vi "Update from Shared Variable.vi"(7 "Force Write (F)":bool, 8 "error in (no error)":errorcluster, 10 "OPC UA server refnum in":refnum<k21>, 11 "SV Sync Tag":refnum<class "Synchronised Tag.lvclass">) -> (0 "error out":errorcluster, 2 "OPC UA server refnum out":refnum<k21>, 3 "SV Sync Tag Out":refnum<class "Synchronised Tag.lvclass">)   [LabVIEW 2016, in "Synchronised Tag.lvclass"]
doc: "Reads the latest value from the shared variable engine and updates the OPC UA server if the value has changed. Use <b>Force Write</b> to write the value whether it has changed or not."
uses:
  Synchronised Tag.lvclass
  Synchronised Tag.lvclass/Synchronised Tag.ctl
  <vilib>/OPCUA/server/Write Double.vi
  <vilib>/OPCUA/server/Write Double Array.vi
  <vilib>/OPCUA/server/Write String.vi
  <vilib>/OPCUA/server/Write String Array.vi
  <vilib>/OPCUA/server/Write Bool.vi
  <vilib>/OPCUA/server/Write Bool Array.vi
  <vilib>/OPCUA/server/Write SByte.vi
  <vilib>/OPCUA/server/Write SByte Array.vi
  <vilib>/OPCUA/server/Write Byte.vi
  <vilib>/OPCUA/server/Write Byte Array.vi
  <vilib>/OPCUA/server/Write Int16.vi
  <vilib>/OPCUA/server/Write Int16 Array.vi
  <vilib>/OPCUA/server/Write UInt16.vi
  <vilib>/OPCUA/server/Write UInt16 Array.vi
  <vilib>/OPCUA/server/Write Int32.vi
  <vilib>/OPCUA/server/Write Int32 Array.vi
  <vilib>/OPCUA/server/Write UInt32.vi
  <vilib>/OPCUA/server/Write UInt32 Array.vi
  <vilib>/OPCUA/server/Write Int64.vi
  <vilib>/OPCUA/server/Write Int64 Array.vi
  <vilib>/OPCUA/server/Write UInt64.vi
  <vilib>/OPCUA/server/Write UInt64 Array.vi
  <vilib>/OPCUA/server/Write Float.vi
  <vilib>/OPCUA/server/Write Float Array.vi
  <vilib>/OPCUA/NI OPC UA Server.lvlib
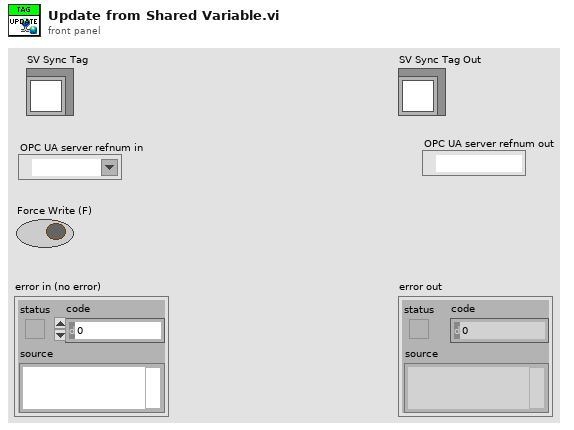
[diagram p1: front panel]
types:
  T1 = typedef "SV type.ctl" = enum16{"Boolean", "SByte", "Byte", "Int16", "UInt16", "Int32", "UInt32", "Int64", "UInt64", "Float", "Double", "String", "DateTime", "ByteString", "Array of Boolean", "Array of SByte", "Array of Byte", "Array of Int16", "Array of UInt16", "Array of Int32", "Array of UInt32", "Array of Int64", "Array of UInt64", "Array of Float", "Array of Double", "Array of String", "Array of DateTime", "Array of ByteString", "Unsupported"}
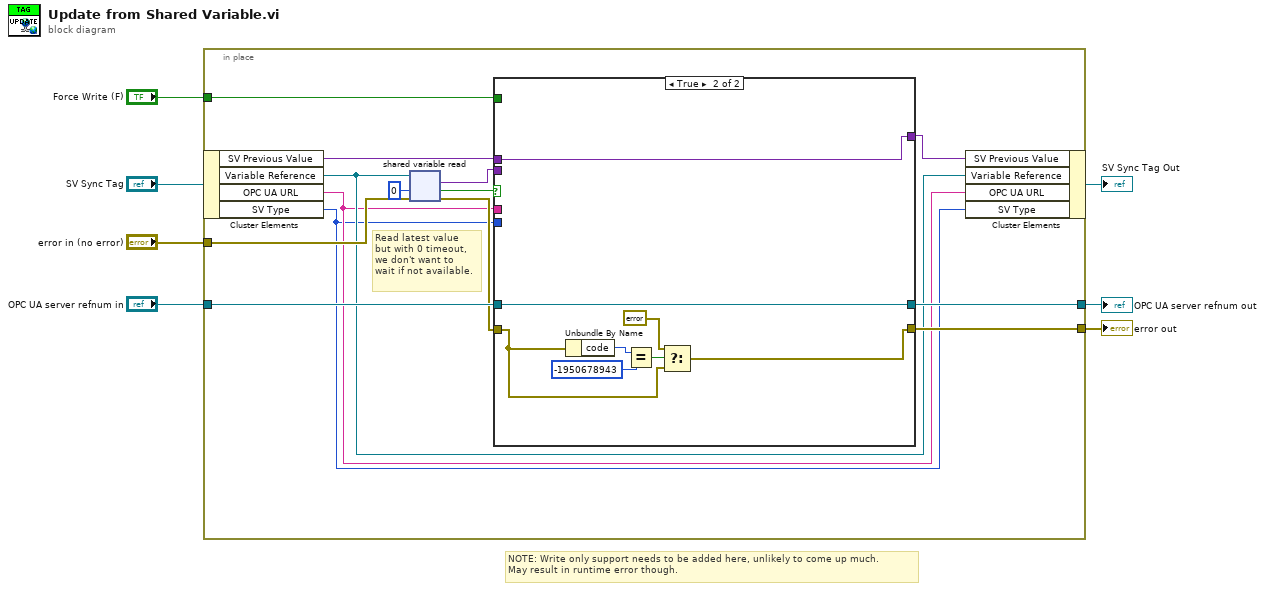
[diagram p0: block diagram]
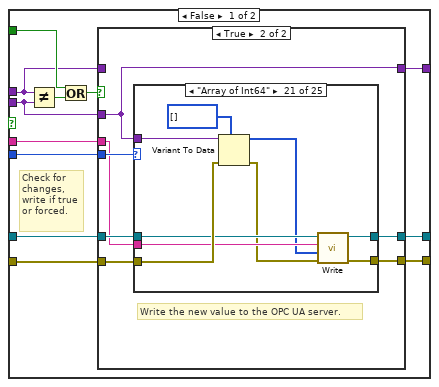
[diagram p2: hidden frame]
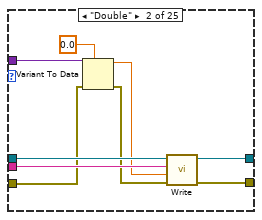
[diagram p5: hidden frame]
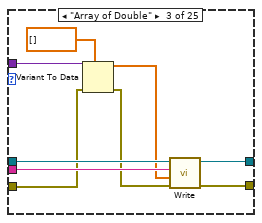
[diagram p6: hidden frame]
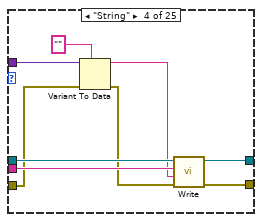
[diagram p7: hidden frame]
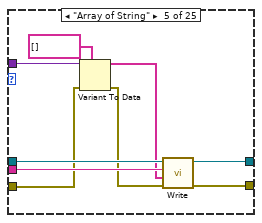
[diagram p8: hidden frame]
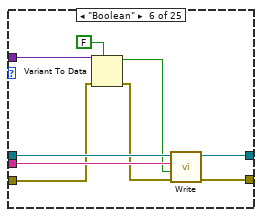
[diagram p9: hidden frame]
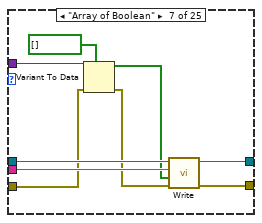
[diagram p10: hidden frame]
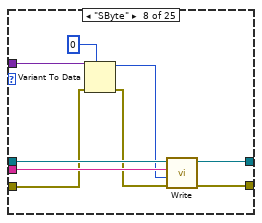
[diagram p11: hidden frame]
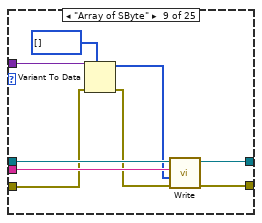
[diagram p12: hidden frame]
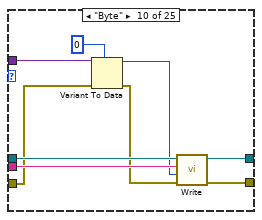
[diagram p13: hidden frame]
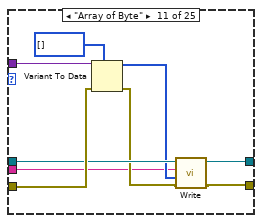
[diagram p14: hidden frame]
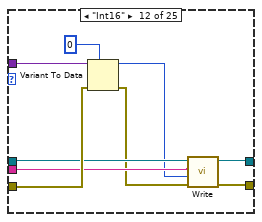
[diagram p15: hidden frame]
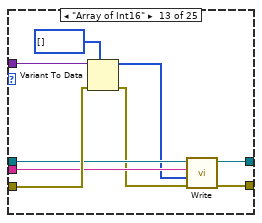
[diagram p16: hidden frame]
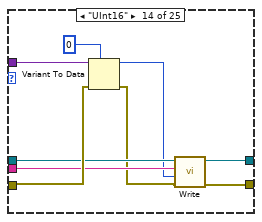
[diagram p17: hidden frame]
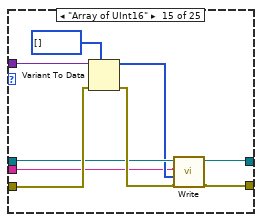
[diagram p18: hidden frame]
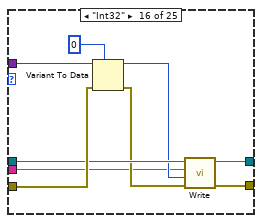
[diagram p19: hidden frame]
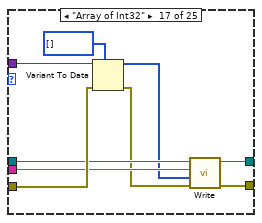
[diagram p20: hidden frame]
diagram:
  # "NOTE: Write only support needs to be added here, unlikely to come up much.\nMay result in runtime error though."
  n1 = in-place {
    in-place-border: "error in (no error)" -> [w21]
    in-place-border: "OPC UA server refnum in" -> [w20]
    in-place-border: [w19] -> w3
    in-place-border: [w18] -> w5
    in-place-border: "Force Write (F)" -> [w17]
    # "Read latest value\nbut with 0 timeout,\nwe don't want to \nwait if not available."
    n2 = in-place-cluster #1("SV Sync Tag") -> ("SV Previous Value"=w12:variant, "Variable Reference"=w10:refnum<k21>, "OPC UA URL"=w9:string, "SV Type"=w8:T1)
    n3 = shared-variable-read(w10, w21, 0 ("timeout ms")) -> (w13:errorcluster, w15:bool, w14:variant)  [unwired: 2 out]
    n4 = case shown="True" w15 {
      tunnel: [w32 w262] -> w11
      tunnel: w14 -> [w25 _]
      tunnel: w12 -> [w22 w262]
      tunnel: w9 -> [w31 _]
      tunnel: w8 -> [w30 _]
      tunnel: w20 -> [w29 w269]
      tunnel: w13 -> [w28 w264]
      tunnel: [w27 w269] -> w18
      tunnel: [w26 w263] -> w19
      tunnel: w17 -> [w23 _]
      frame False {
        # "Check for\nchanges,\nwrite if true\nor forced."
        n5 = Not Equal?(x=w22, y=w25) -> (x != y?=w33:bool)
        n6 = Or(x=w23, y=w33) -> (x .or. y?=w24:bool)
        n7 = case shown="True" w24 {
          tunnel: [w34 w37] -> w32
          tunnel: w31 -> [_ w41]
          tunnel: w30 -> [_ w43]
          tunnel: w29 -> [w36 w42]
          tunnel: w28 -> [w35 w40]
          tunnel: [w36 w39] -> w27
          tunnel: [w35 w38] -> w26
          tunnel: w25 -> [_ w37]
          tunnel: w22 -> [w34 _]
          frame False {
          }
          frame True {
            # "Write the new value to the OPC UA server."
            n8 = case shown="\"Array of Int64\"" w43 {
              tunnel: w37 -> [_ w54 w63 w72 w81 w90 w99 w108 w117 w126 w135 w144 w153 w162 w171 w180 w189 w198 w207 w216 w225 w234 w243 w252 w261]
              tunnel: w42 -> [w45 w51 w61 w69 w78 w87 w98 w105 w116 w123 w130 w139 w148 w157 w165 w175 w184 w193 w202 w211 w220 w229 w238 w247 w256]
              tunnel: [w45 w53 w62 w71 w80 w89 w97 w107 w115 w124 w132 w140 w149 w159 w167 w176 w185 w194 w203 w212 w221 w230 w239 w246 w257] -> w39
              tunnel: w40 -> [w44 w48 w57 w65 w74 w83 w92 w102 w111 w120 w133 w142 w151 w160 w169 w178 w187 w196 w205 w214 w223 w232 w241 w250 w259]
              tunnel: [w44 w52 w60 w70 w79 w88 w96 w106 w114 w125 w131 w141 w150 w158 w168 w177 w186 w195 w204 w213 w222 w231 w240 w249 w258] -> w38
              tunnel: w41 -> [_ w50 w59 w68 w77 w86 w95 w104 w113 w122 w127 w138 w147 w156 w163 w172 w183 w192 w201 w210 w219 w228 w237 w245 w253]
              frame Default {
              }
              frame "Double" {
                n9 = Variant To Data(error in=w48, type=0.0 ("value"), Variant=w54) -> (data=w46:dbl, error out=w47:errorcluster)
                n10 = call-poly <vilib>:"Write.vi"("error in (no error)"=w47, "value"=w46, "node path"=w50, "OPC UA server refnum in"=w51) -> ("error out"=w52:errorcluster, "OPC UA server refnum out"=w53:refnum<k21>)  [unwired: 6 in]
              }
              frame "Array of Double" {
                n11 = Variant To Data(error in=w57, type=dbl[] [] ("value"), Variant=w63) -> (data=w55:dbl[], error out=w56:errorcluster)
                n12 = call-poly <vilib>:"Write.vi"("error in (no error)"=w56, "value"=w55, "node path"=w59, "OPC UA server refnum in"=w61) -> ("error out"=w60:errorcluster, "OPC UA server refnum out"=w62:refnum<k21>)  [unwired: 6 in]
              }
              frame "String" {
                n13 = Variant To Data(error in=w65, type="" ("name"), Variant=w72) -> (data=w67:string, error out=w64:errorcluster)
                n14 = call-poly <vilib>:"Write.vi"("error in (no error)"=w64, "value"=w67, "node path"=w68, "OPC UA server refnum in"=w69) -> ("error out"=w70:errorcluster, "OPC UA server refnum out"=w71:refnum<k21>)  [unwired: 6 in]
              }
              frame "Array of String" {
                n15 = Variant To Data(error in=w74, type=string[] [] ("value"), Variant=w81) -> (data=w75:string[], error out=w73:errorcluster)
                n16 = call-poly <vilib>:"Write.vi"("error in (no error)"=w73, "value"=w75, "node path"=w77, "OPC UA server refnum in"=w78) -> ("error out"=w79:errorcluster, "OPC UA server refnum out"=w80:refnum<k21>)  [unwired: 6 in]
              }
              frame "Boolean" {
                n17 = Variant To Data(error in=w83, type=FALSE ("value"), Variant=w90) -> (data=w84:bool, error out=w82:errorcluster)
                n18 = call-poly <vilib>:"Write.vi"("error in (no error)"=w82, "value"=w84, "node path"=w86, "OPC UA server refnum in"=w87) -> ("error out"=w88:errorcluster, "OPC UA server refnum out"=w89:refnum<k21>)  [unwired: 6 in]
              }
              frame "Array of Boolean" {
                n19 = Variant To Data(error in=w92, type=bool[] [] ("value"), Variant=w99) -> (data=w93:bool[], error out=w91:errorcluster)
                n20 = call-poly <vilib>:"Write.vi"("error in (no error)"=w91, "value"=w93, "node path"=w95, "OPC UA server refnum in"=w98) -> ("error out"=w96:errorcluster, "OPC UA server refnum out"=w97:refnum<k21>)  [unwired: 6 in]
              }
              frame "SByte" {
                n21 = Variant To Data(error in=w102, type=i8 0 ("value"), Variant=w108) -> (data=w100:i8, error out=w101:errorcluster)
                n22 = call-poly <vilib>:"Write.vi"("error in (no error)"=w101, "value"=w100, "node path"=w104, "OPC UA server refnum in"=w105) -> ("error out"=w106:errorcluster, "OPC UA server refnum out"=w107:refnum<k21>)  [unwired: 6 in]
              }
              frame "Array of SByte" {
                n23 = Variant To Data(error in=w111, type=i8[] [] ("value"), Variant=w117) -> (data=w109:i8[], error out=w110:errorcluster)
                n24 = call-poly <vilib>:"Write.vi"("error in (no error)"=w110, "value"=w109, "node path"=w113, "OPC UA server refnum in"=w116) -> ("error out"=w114:errorcluster, "OPC UA server refnum out"=w115:refnum<k21>)  [unwired: 6 in]
              }
              frame "Byte" {
                n25 = Variant To Data(error in=w120, type=u8 0 ("value"), Variant=w126) -> (data=w118:u8, error out=w119:errorcluster)
                n26 = call-poly <vilib>:"Write.vi"("error in (no error)"=w119, "value"=w118, "node path"=w122, "OPC UA server refnum in"=w123) -> ("error out"=w125:errorcluster, "OPC UA server refnum out"=w124:refnum<k21>)  [unwired: 6 in]
              }
              frame "Array of Byte" {
                n27 = Variant To Data(error in=w133, type=u8[] [] ("value"), Variant=w135) -> (data=w128:u8[], error out=w129:errorcluster)
                n28 = call-poly <vilib>:"Write.vi"("error in (no error)"=w129, "value"=w128, "node path"=w127, "OPC UA server refnum in"=w130) -> ("error out"=w131:errorcluster, "OPC UA server refnum out"=w132:refnum<k21>)  [unwired: 6 in]
              }
              frame "Int16" {
                n29 = Variant To Data(error in=w142, type=i16 0 ("value"), Variant=w144) -> (data=w136:i16, error out=w137:errorcluster)
                n30 = call-poly <vilib>:"Write.vi"("error in (no error)"=w137, "value"=w136, "node path"=w138, "OPC UA server refnum in"=w139) -> ("error out"=w141:errorcluster, "OPC UA server refnum out"=w140:refnum<k21>)  [unwired: 6 in]
              }
              frame "Array of Int16" {
                n31 = Variant To Data(error in=w151, type=i16[] [] ("value"), Variant=w153) -> (data=w146:i16[], error out=w145:errorcluster)
                n32 = call-poly <vilib>:"Write.vi"("error in (no error)"=w145, "value"=w146, "node path"=w147, "OPC UA server refnum in"=w148) -> ("error out"=w150:errorcluster, "OPC UA server refnum out"=w149:refnum<k21>)  [unwired: 6 in]
              }
              frame "UInt16" {
                n33 = Variant To Data(error in=w160, type=u16 0 ("value"), Variant=w162) -> (data=w154:u16, error out=w155:errorcluster)
                n34 = call-poly <vilib>:"Write.vi"("error in (no error)"=w155, "value"=w154, "node path"=w156, "OPC UA server refnum in"=w157) -> ("error out"=w158:errorcluster, "OPC UA server refnum out"=w159:refnum<k21>)  [unwired: 6 in]
              }
              frame "Array of UInt16" {
                n35 = Variant To Data(error in=w169, type=u16[] [] ("value"), Variant=w171) -> (data=w164:u16[], error out=w166:errorcluster)
                n36 = call-poly <vilib>:"Write.vi"("error in (no error)"=w166, "value"=w164, "node path"=w163, "OPC UA server refnum in"=w165) -> ("error out"=w168:errorcluster, "OPC UA server refnum out"=w167:refnum<k21>)  [unwired: 6 in]
              }
              frame "Int32" {
                n37 = Variant To Data(error in=w178, type=0 ("value"), Variant=w180) -> (data=w173:i32, error out=w174:errorcluster)
                n38 = call-poly <vilib>:"Write.vi"("error in (no error)"=w174, "value"=w173, "node path"=w172, "OPC UA server refnum in"=w175) -> ("error out"=w177:errorcluster, "OPC UA server refnum out"=w176:refnum<k21>)  [unwired: 6 in]
              }
              frame "Array of Int32" {
                n39 = Variant To Data(error in=w187, type=i32[] [] ("value"), Variant=w189) -> (data=w182:i32[], error out=w181:errorcluster)
                n40 = call-poly <vilib>:"Write.vi"("error in (no error)"=w181, "value"=w182, "node path"=w183, "OPC UA server refnum in"=w184) -> ("error out"=w186:errorcluster, "OPC UA server refnum out"=w185:refnum<k21>)  [unwired: 6 in]
              }
              frame "UInt32" {
                n41 = Variant To Data(error in=w196, type=u32 0 ("value"), Variant=w198) -> (data=w191:u32, error out=w190:errorcluster)
                n42 = call-poly <vilib>:"Write.vi"("error in (no error)"=w190, "value"=w191, "node path"=w192, "OPC UA server refnum in"=w193) -> ("error out"=w195:errorcluster, "OPC UA server refnum out"=w194:refnum<k21>)  [unwired: 6 in]
              }
              frame "Array of UInt32" {
                n43 = Variant To Data(error in=w205, type=u32[] [] ("value"), Variant=w207) -> (data=w200:u32[], error out=w199:errorcluster)
                n44 = call-poly <vilib>:"Write.vi"("error in (no error)"=w199, "value"=w200, "node path"=w201, "OPC UA server refnum in"=w202) -> ("error out"=w204:errorcluster, "OPC UA server refnum out"=w203:refnum<k21>)  [unwired: 6 in]
              }
              frame "Int64" {
                n45 = Variant To Data(error in=w214, type=i64 0 ("value"), Variant=w216) -> (data=w209:i64, error out=w208:errorcluster)
                n46 = call-poly <vilib>:"Write.vi"("error in (no error)"=w208, "value"=w209, "node path"=w210, "OPC UA server refnum in"=w211) -> ("error out"=w213:errorcluster, "OPC UA server refnum out"=w212:refnum<k21>)  [unwired: 6 in]
              }
              frame "Array of Int64" {
                n47 = Variant To Data(error in=w223, type=i64[] [] ("value"), Variant=w225) -> (data=w218:i64[], error out=w217:errorcluster)
                n48 = call-poly <vilib>:"Write.vi"("error in (no error)"=w217, "value"=w218, "node path"=w219, "OPC UA server refnum in"=w220) -> ("error out"=w222:errorcluster, "OPC UA server refnum out"=w221:refnum<k21>)  [unwired: 6 in]
              }
              frame "UInt64" {
                n49 = Variant To Data(error in=w232, type=u64 0 ("value"), Variant=w234) -> (data=w226:u64, error out=w227:errorcluster)
                n50 = call-poly <vilib>:"Write.vi"("error in (no error)"=w227, "value"=w226, "node path"=w228, "OPC UA server refnum in"=w229) -> ("error out"=w231:errorcluster, "OPC UA server refnum out"=w230:refnum<k21>)  [unwired: 6 in]
              }
              frame "Array of UInt64" {
                n51 = Variant To Data(error in=w241, type=u64[] [] ("value"), Variant=w243) -> (data=w236:u64[], error out=w235:errorcluster)
                n52 = call-poly <vilib>:"Write.vi"("error in (no error)"=w235, "value"=w236, "node path"=w237, "OPC UA server refnum in"=w238) -> ("error out"=w240:errorcluster, "OPC UA server refnum out"=w239:refnum<k21>)  [unwired: 6 in]
              }
              frame "Float" {
                n53 = Variant To Data(error in=w250, type=sgl 0.0 ("value"), Variant=w252) -> (data=w244:sgl, error out=w248:errorcluster)
                n54 = call-poly <vilib>:"Write.vi"("error in (no error)"=w248, "value"=w244, "node path"=w245, "OPC UA server refnum in"=w247) -> ("error out"=w249:errorcluster, "OPC UA server refnum out"=w246:refnum<k21>)  [unwired: 6 in]
              }
              frame "Array of Float" {
                n55 = Variant To Data(error in=w259, type=sgl[] [] ("value"), Variant=w261) -> (data=w254:sgl[], error out=w255:errorcluster)
                n56 = call-poly <vilib>:"Write.vi"("error in (no error)"=w255, "value"=w254, "node path"=w253, "OPC UA server refnum in"=w256) -> ("error out"=w258:errorcluster, "OPC UA server refnum out"=w257:refnum<k21>)  [unwired: 6 in]
              }
            }
          }
        }
      }
      frame True {
        n57 = Unbundle By Name(w264) -> ("code"=w268:i32)
        n58 = Equal?(x=w268, y=-1950678943) -> (x = y?=w266:bool)
        n59 = Select(t=errorcluster {"status"=FALSE, "code"=0, "source"=""}, s=w266, f=w264) -> (s? t:f=w263:errorcluster)
      }
    }
    n60 = in-place-cluster #1("SV Previous Value"=w11, "Variable Reference"=w10, "OPC UA URL"=w9, "SV Type"=w8) -> (→"SV Sync Tag Out":refnum<class "Synchronised Tag.lvclass">)
  }
  "error out" <- w3
  "OPC UA server refnum out" <- w5
